vi "FTW-Test-JSON-ObjectDelete.vi"() -> (0 "Test Result":errorcluster)   [LabVIEW 2015]
panel:
  out "Original JSON":string
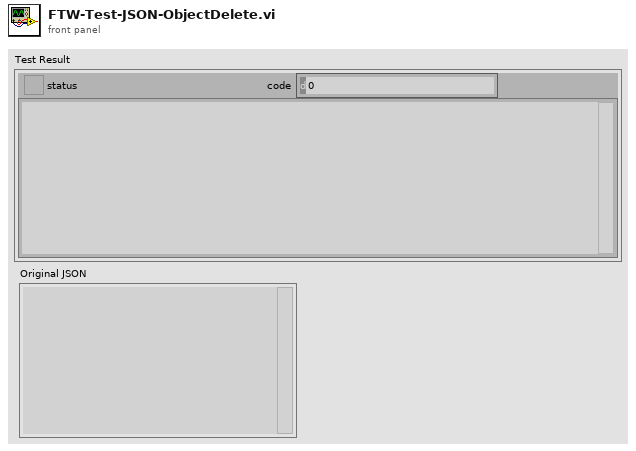
[diagram p1: front panel]
types:
  T1 = typedef "FTW-Type-JSON.ctl" = refnum<data-value>
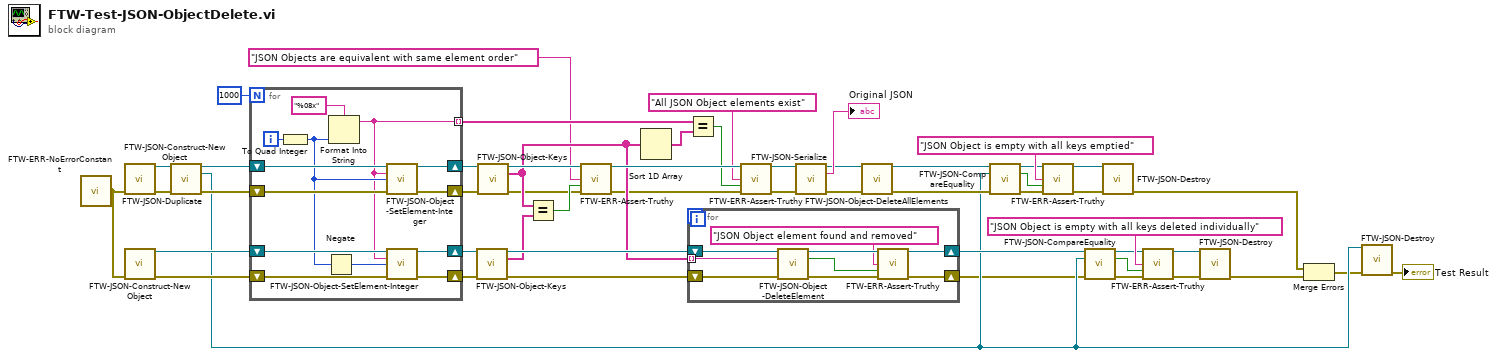
[diagram p0: block diagram]
diagram:
  n1 = call "FTW-ERR-NoErrorConstant.vi"() -> ("no error"=w46:errorcluster)
  n2 = call "FTW-JSON-Construct-NewObject.vi"("error in"=w46) -> ("JSON"=w43:T1, "error out"=w42:errorcluster)  [unwired: 13 in]
  n3 = call "FTW-JSON-Construct-NewObject.vi"("error in"=w46) -> ("JSON"=w44:T1, "error out"=w45:errorcluster)  [unwired: 13 in]
  n4 = call "FTW-JSON-Duplicate.vi"("JSON"=w43, "error in"=w42) -> ("JSON out"=w40:T1, "Duplicated JSON"=w17:T1, "error out"=w41:errorcluster)  [unwired: 11 in]
  n5 = for {
    N: 1000 -> [_]
    shift-right: [w58] -> w37
    shift-left: w41 -> [w59]
    shift-right: [w60] -> w39
    shift-left: w40 -> [w61]
    shift-right: [w53] -> w9
    shift-left: w45 -> [w55]
    shift-right: [w54] -> w10
    shift-left: w44 -> [w56]
    tunnel: [w49] -> w35 mode=indexing
    i -> [w57]
    n6 = To Quad Integer(1:w57) -> (0:w50:i64)
    n7 = Negate(x=w50) -> (-x=w51:i64)
    n8 = Format Into String(format string="%08x", w50) -> (resulting string=w49:string)  [unwired: 2 in, 1 out]
    n9 = call "FTW-JSON-Object-SetElement-Integer.vi"("JSON"=w61, "Key"=w49, "Value"=w50, "error in"=w59) -> ("JSON out"=w60:T1, "error out"=w58:errorcluster)  [unwired: 10 in]
    n10 = call "FTW-JSON-Object-SetElement-Integer.vi"("JSON"=w56, "Key"=w49, "Value"=w51, "error in"=w55) -> ("JSON out"=w54:T1, "error out"=w53:errorcluster)  [unwired: 10 in]
  }
  n11 = call "FTW-JSON-Object-Keys.vi"("JSON"=w10, "error in"=w9) -> ("JSON out"=w8:T1, "Keys"=w6:string[], "error out"=w2:errorcluster)  [unwired: 11 in]
  n12 = call "FTW-JSON-Object-Keys.vi"("JSON"=w39, "error in"=w37) -> ("JSON out"=w38:T1, "Keys"=w7:string[], "error out"=w4:errorcluster)  [unwired: 11 in]
  n13 = Equal?(x=w7, y=w6) -> (x = y?=w5:bool)
  n14 = call "FTW-ERR-Assert-Truthy.vi"("Assertion"="JSON Objects are equivalent with same element order", "Assertion holds true?"=w5, "error in"=w4) -> ("error out"=w3:errorcluster)  [unwired: 12 in]
  n15 = Sort 1D Array(array=w7) -> (sorted array=w36:string[])
  n16 = Equal?(x=w35, y=w36) -> (x = y?=w26:bool)
  n17 = for {
    shift-right: [w66] -> w18
    shift-left: w8 -> [w69]
    shift-right: [w64] -> w13
    shift-left: w2 -> [w68]
    tunnel: w7 -> [w67] mode=indexing
    n18 = call "FTW-JSON-Object-DeleteElement.vi"("JSON"=w69, "Key"=w67, "error in"=w68) -> ("JSON out"=w66:T1, "Found and Removed?"=w63:bool, "error out"=w65:errorcluster)  [unwired: 10 in]
    n19 = call "FTW-ERR-Assert-Truthy.vi"("Assertion"="JSON Object element found and removed", "Assertion holds true?"=w63, "error in"=w65) -> ("error out"=w64:errorcluster)  [unwired: 12 in]
  }
  n20 = call "FTW-ERR-Assert-Truthy.vi"("Assertion"="All JSON Object elements exist", "Assertion holds true?"=w26, "error in"=w3) -> ("error out"=w27:errorcluster)  [unwired: 12 in]
  n21 = call "FTW-JSON-Serialize.vi"("JSON"=w38, "error in"=w27) -> ("JSON out"=w34:T1, "JSON String (UTF-8)"=→"Original JSON":string, "error out"=w33:errorcluster)  [unwired: 11 in]
  n22 = call "FTW-JSON-Object-DeleteAllElements.vi"("JSON"=w34, "error in"=w33) -> ("JSON out"=w24:T1, "error out"=w22:errorcluster)  [unwired: 12 in]
  n23 = call "FTW-JSON-CompareEquality.vi"("JSON"=w24, "JSON to Compare"=w17, "error in"=w22) -> ("JSON out"=w23:T1, "Equal?"=w31:bool, "error out"=w21:errorcluster)  [unwired: 10 in]
  n24 = call "FTW-ERR-Assert-Truthy.vi"("Assertion"="JSON Object is empty with all keys emptied", "Assertion holds true?"=w31, "error in"=w21) -> ("error out"=w20:errorcluster)  [unwired: 12 in]
  n25 = call "FTW-JSON-CompareEquality.vi"("JSON"=w18, "JSON to Compare"=w17, "error in"=w13) -> ("JSON out"=w19:T1, "Equal?"=w29:bool, "error out"=w14:errorcluster)  [unwired: 10 in]
  n26 = call "FTW-JSON-Destroy.vi"("JSON"=w23, "error in"=w20) -> ("error out"=w16:errorcluster)  [unwired: 13 in]
  n27 = call "FTW-ERR-Assert-Truthy.vi"("Assertion"="JSON Object is empty with all keys deleted individually", "Assertion holds true?"=w29, "error in"=w14) -> ("error out"=w28:errorcluster)  [unwired: 12 in]
  n28 = call "FTW-JSON-Destroy.vi"("JSON"=w19, "error in"=w28) -> ("error out"=w15:errorcluster)  [unwired: 13 in]
  n29 = Merge Errors(w16, w15) -> (w12:errorcluster)
  n30 = call "FTW-JSON-Destroy.vi"("JSON"=w17, "error in"=w12) -> ("error out"=→"Test Result":errorcluster)  [unwired: 13 in]
